vi "Autonomous Independent.vi"() -> ()   [LabVIEW 2012]
doc: "This VI is called when autonomous begins, and will automatically be terminated when autonomous ends. You can carry out timed or sensor driven robot movement independently without needing to return to the caller."
uses:
  <vilib>/Rock Robotics/WPI/RobotDrive/WPI_RobotDriveGetSetRefNum.vi
  Robot Global Data.vi
panel:
  out "Shooter Angle Good":bool
  out "Shooter Angle":T1(ring)
  out "Shooter Speed":T2(ring)
  out "Stop Drive":bool
  out "Shift Low":bool
  out "Feeder Happy":bool
  out "Auton Done":bool
  out "Shooter Happy":bool
  out "Shoot!":bool
  out "Delay Switch":u32
  out "Seccond Switch":u32
  out "First Switch":u32
  # "Be sure to right-click and choose Data Operations>>Make Current Value default if you want to save the array values with the VI"
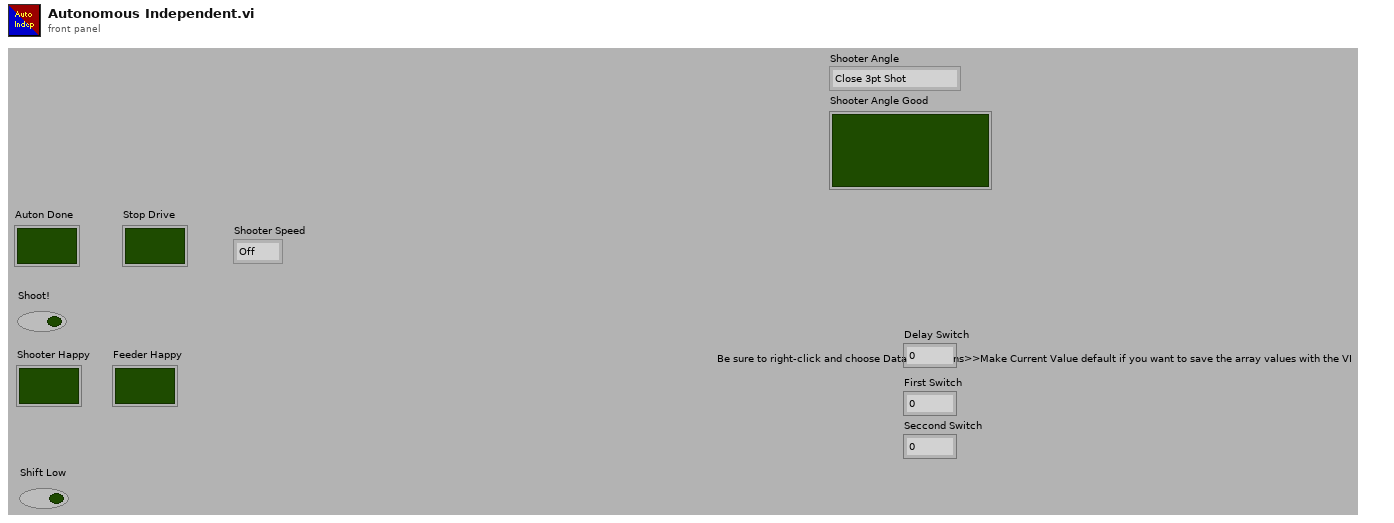
[diagram p1: front panel]
types:
  T1 = enum16{"Close 3pt Shot", "Far 3pt Shot", "Feeding"}
  T2 = enum16{"Off", "Close Pyramid 3pt", "Far Pyramid 3pt", "Feeder Shot", "UD Far 3pt Shot"}
  T3 = enum16{"Off", "Close Pyramid 3pt", "Far Pyramid 3pt", "Feeder Shot"}
  T4 = typedef "WPI_RobotDriveDevRef.ctl" = cluster{"DevStatus":errorcluster, "Motors[]":T5[], "Square Inputs":bool, "Max Output":dbl, "Isochronous":bool}
  T5 = typedef "WPI_MotorControlDeviceRef.ctl" = cluster{"DeviceStatus":errorcluster, "Type":enum16{"PWM", "CAN"}, "PWM":cluster{"Digital Module":T6, "PWM Channel":T7, "DeadBand":T8}, "CAN":cluster{"Device Number":u8, "Control Mode":T9, "Semaphore":T10, "Max Vout":dbl}, "Invert":bool, "TransformRef":T11, "InvTransformRef":T11}
  T6 = typedef "FPGA_TypedefDigitalModule.ctl" = enum16{"Digital Module 1", "Digital Module 2"}
  T7 = typedef "FPGA_DIOPWMChannel.ctl" = enum8{"PWM 1", "PWM 2", "PWM 3", "PWM 4", "PWM 5", "PWM 6", "PWM 7", "PWM 8", "PWM 9", "PWM 10", "Invalid"}
  T8 = typedef "WPI_PWMDeadband.ctl" = cluster{"Name":string, "maxPositivePwm":i32, "minPositivePwm":i32, "centerPwm":i32, "maxNegativePwm":i32, "minNegativePwm":i32, "angularRange":u16}
  T9 = typedef "WPI_CANJaguar_ControlMode.ctl" = enum8{"Percent VBus", "Current", "Speed", "Position", "Voltage"}
  T10 = typedef "Semaphore RefNum" = refnum<k1>
  T11 = typedef "WPI_PWMTransform_ConPane.ctl" = refnum<vi>
  T12 = typedef "WPI_GyroDevRef.ctl" = cluster{"DevStatus":errorcluster, "Analog Module":T13, "Analog Channel":T14, "Offset":dbl, "Gain (VoltsPerDegree/Second)":dbl}
  T13 = typedef "FPGA_TypedefAnalogModule.ctl" = enum16{"Analog Module 1", "Analog Module 2"}
  T14 = typedef "FPGA_AIChannel.ctl" = enum8{"AI 1", "AI 2", "AI 3", "AI 4", "AI 5", "AI 6", "AI 7", "AI 8", "Invalid"}
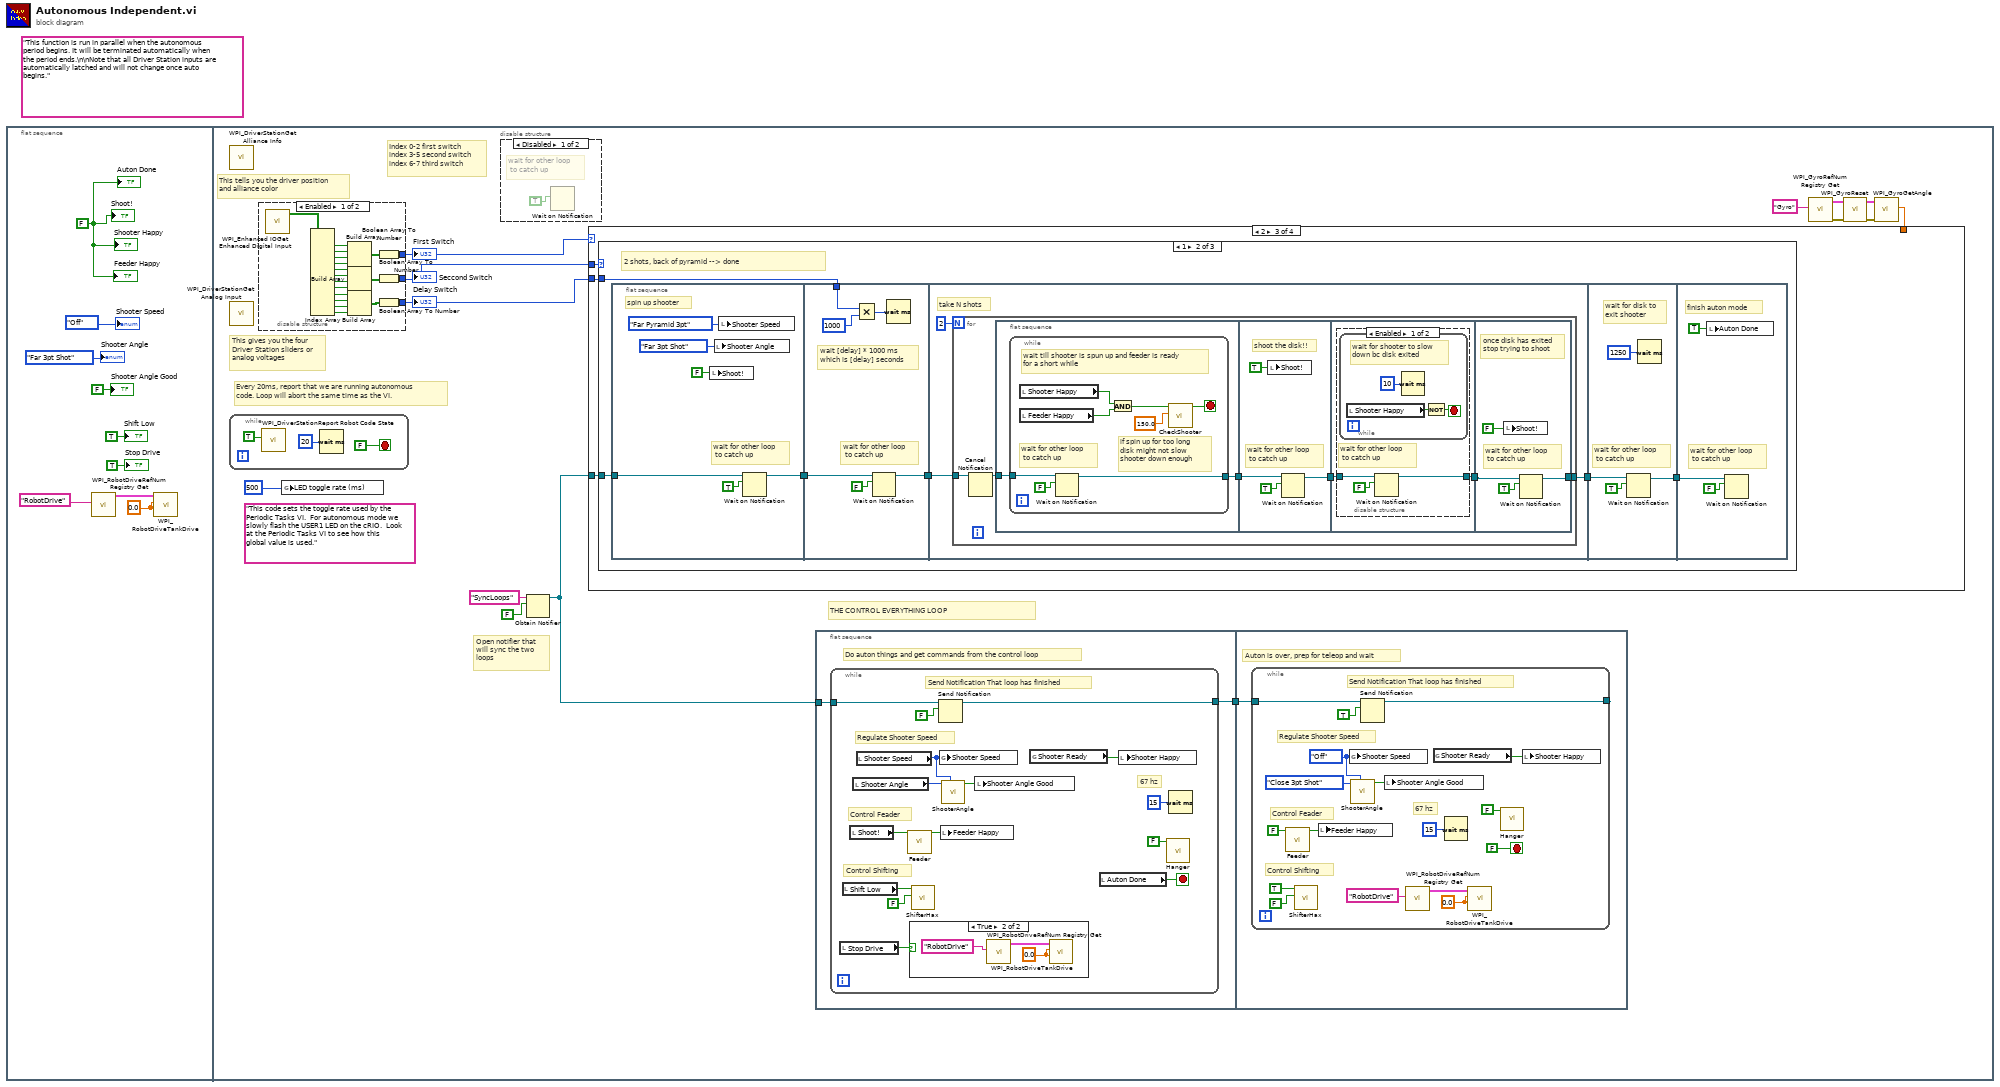
[diagram p0: block diagram]
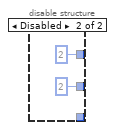
[diagram p2: hidden frame]
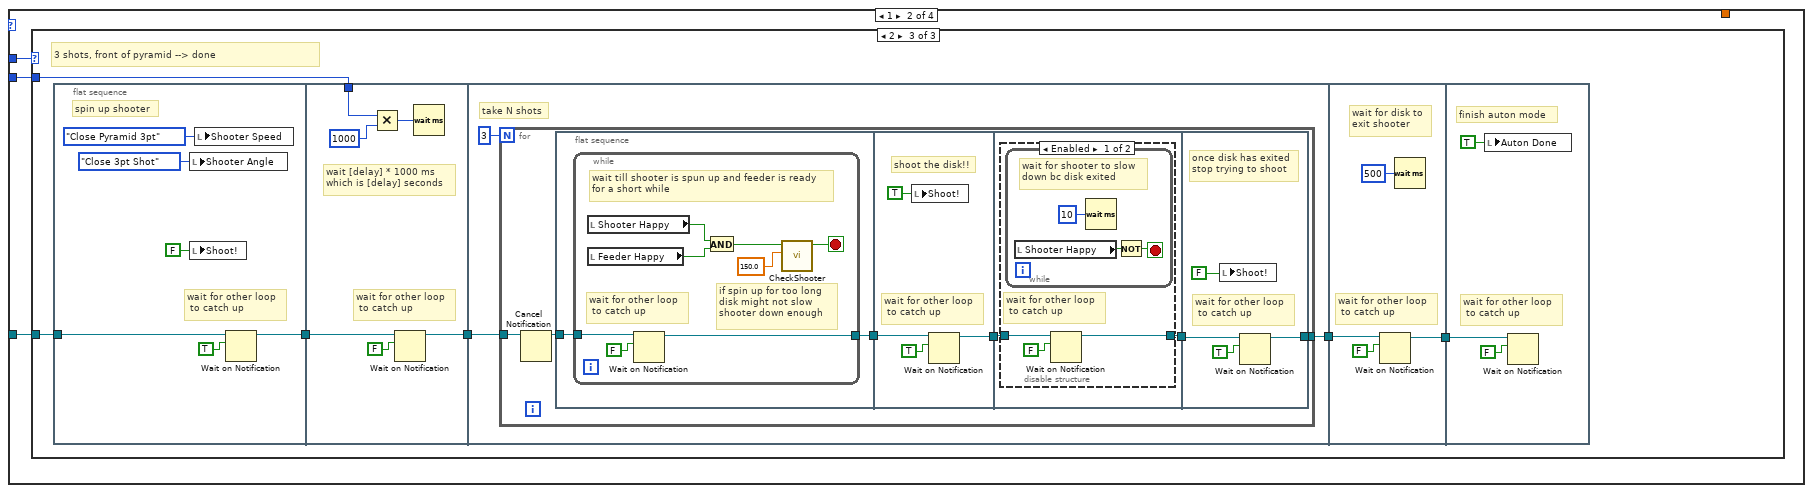
[diagram p6: hidden frame]
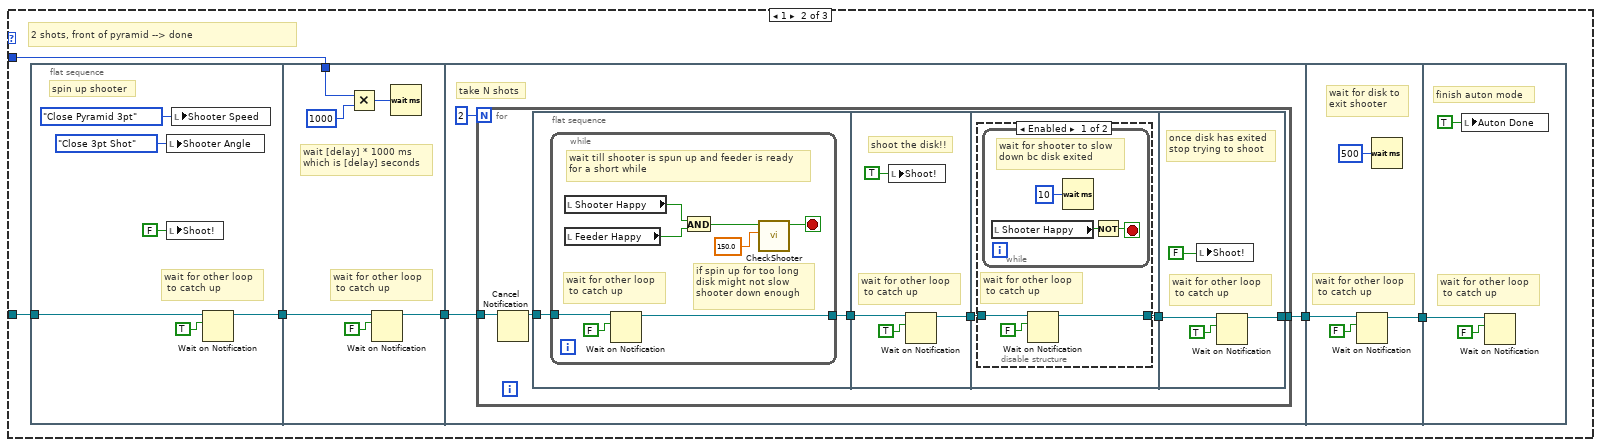
[diagram p8: hidden frame]
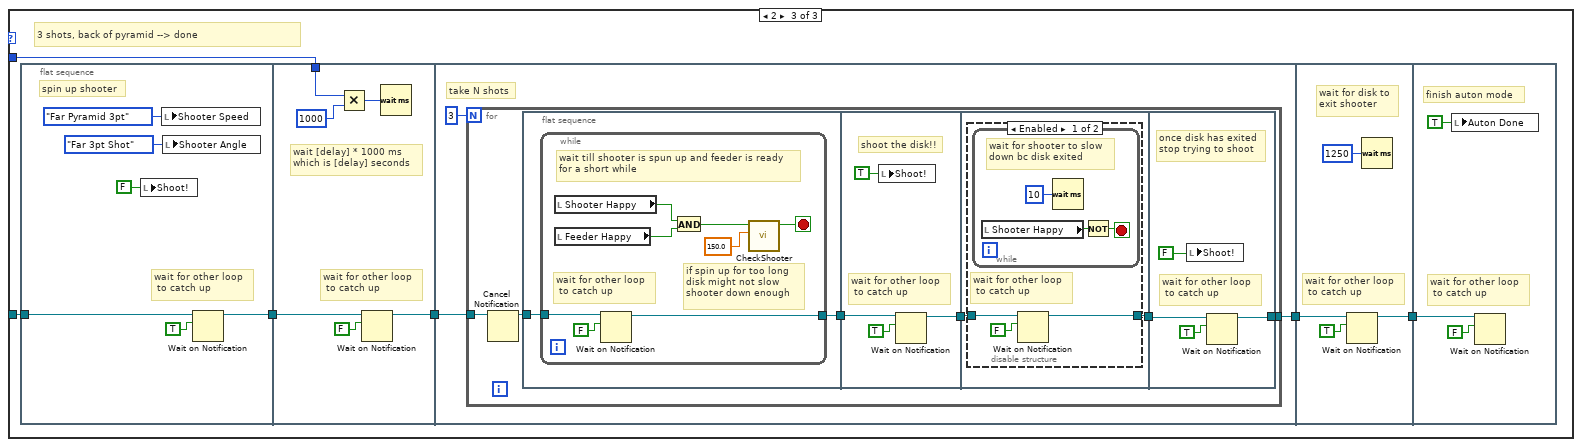
[diagram p13: hidden frame]
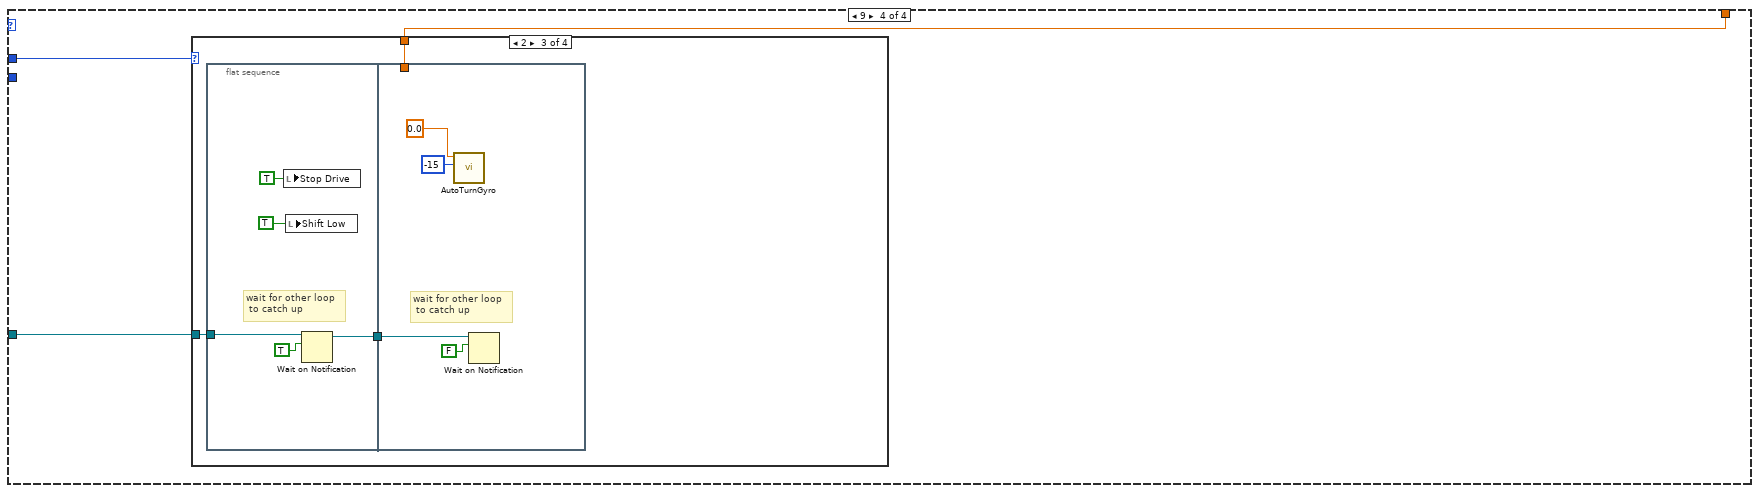
[diagram p15: hidden frame]
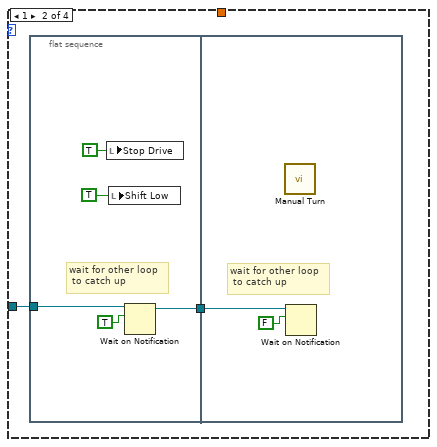
[diagram p17: hidden frame]
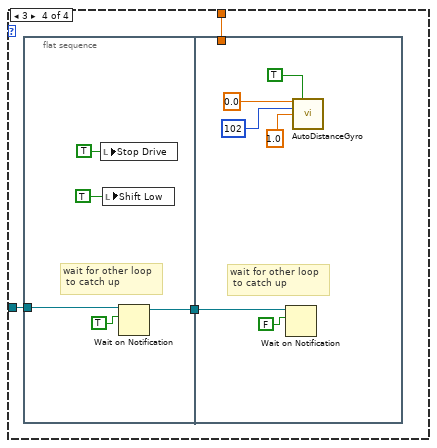
[diagram p18: hidden frame]
diagram:
  (unwired) "This function is run in parallel when the autonomous period begins. It will be terminated automatically when the period ends.\n\nNote that all Driver Station inputs are automatically latched and will not change once auto begins."
  n1 = flat-sequence {
    frame #0 {
      w5 = 0.0 ("Left axis value")
      w9 = FALSE
      n2 = call <vilib>:"WPI_RobotDriveRefNum Registry Get.vi"("refnum name"="RobotDrive") -> ("RobotDriveDevRef"=w6:T4)  [unwired: 1 in, 9 out]
      n3 = call <vilib>:"WPI_RobotDriveTankDrive.vi"("Right axis value"=w5, "Left axis value"=w5, "RobotDriveDevRef"=w6) -> ()  [unwired: 6 in, 3 out]
      "Feeder Happy" <- w9
      "Shift Low" <- TRUE ("Shift Low")
      "Stop Drive" <- TRUE ("Stop Drive")
      "Shoot!" <- w9
      "Shooter Happy" <- w9
      "Auton Done" <- w9
      "Shooter Speed" <- T3."Off" ("Shooter Speed")
      "Shooter Angle" <- T1."Far 3pt Shot" ("Target Shooter Angle")
      "Shooter Angle Good" <- FALSE ("Shooter Angle Good")
    }
    frame #1 {
      (unwired) "This code sets the toggle rate used by the Periodic Tasks VI.  For autonomous mode we slowly flash the USER1 LED on the cRIO.  Look at the Periodic Tasks VI to see how this global value is used."
      # "THE CONTROL EVERYTHING LOOP"
      # "Index 0-2 first switch\nindex 3-5 second switch\nindex 6-7 third switch"
      # "Open notifier that\nwill sync the two\nloops"
      # "Every 20ms, report that we are running autonomous\ncode. Loop will abort the same time as the VI."
      # "This tells you the driver position\nand alliance color"
      # "This gives you the four\nDriver Station sliders or\nanalog voltages"
      n4 = call <vilib>:"WPI_DriverStationGet Alliance Info.vi"() -> ()  [unwired: 12 out]
      n5 = call <vilib>:"WPI_DriverStationGet Analog Input.vi"() -> ()  [unwired: 12 out]
      n6 = while {
        stop <- FALSE stop-if-true
        n7 = call <vilib>:"WPI_DriverStationReport Robot Code State.vi"("Autonomous"=TRUE) -> ()  [unwired: 10 in, 1 out]
        n8 = Wait (ms)(milliseconds to wait=u32 20) -> ()  [unwired: 1 out]
      }
      n9 = disable-structure shown="Enabled" {
        disable-tunnel: [w26 u32 2 ("First Switch")] -> w18
        disable-tunnel: [w25 u32 2 ("Seccond Switch")] -> w17
        disable-tunnel: [w24 _] -> w15
        frame Enabled {
          n10 = call <vilib>:"WPI_Enhanced IOGet Enhanced Digital Input.vi"() -> ("Digital Input [1-16]"=w27:bool[])  [unwired: 10 in, 1 out]
          n11 = Index Array(array=w27) -> (element #1=w42:bool, element #2=w41:bool, element #3=w40:bool, element #4=w33:bool, element #5=w39:bool, element #6=w38:bool, element #7=w35:bool, element #8=w34:bool, element #9=w32:bool, element #10=w31:bool, element #11=w30:bool, element #12=w29:bool)  [unwired: 12 in]
          n12 = Build Array(w42, w41, w40, w33) -> (w36:bool[])
          n13 = Build Array(w39, w38, w35, w34) -> (w37:bool[])
          n14 = Build Array(w32, w31, w30, w29) -> (w28:bool[])
          n15 = Boolean Array To Number(Boolean array=w36) -> (number=w26:u32)
          n16 = Boolean Array To Number(Boolean array=w37) -> (number=w25:u32)
          n17 = Boolean Array To Number(Boolean array=w28) -> (number=w24:u32)
        }
        frame Disabled {
        }
      }
      "First Switch" <- w18
      "Seccond Switch" <- w17
      "Delay Switch" <- w15
      n18 = global write "Robot Global Data.vi" "LED toggle rate (ms)"(u32 500 ("LED ms toggle rate")) -> ()
      n19 = disable-structure shown="Disabled" {
        frame Disabled {
          # "wait for other loop\n to catch up"
          n20 = Wait on Notification(ignore previous (F)=TRUE) -> (notifier=w46:refnum<notifier>)  [unwired: 2 in, 4 out]
        }
        frame Enabled {
        }
      }
      n21 = Obtain Notifier(name (unnamed)="SyncLoops", notification data type=FALSE) -> (notifier out=w16:refnum<notifier>)  [unwired: 2 in, 2 out]
      n22 = flat-sequence {
        tunnel: w16 -> [w48]
        tunnel: [w47] -> w23
        tunnel: w23 -> [w67]
        frame #0 {
          # "Do auton things and get commands from the control loop"
          n23 = while {
            tunnel: w48 -> [w61]
            tunnel: [w59] -> w47
            stop <- w63 stop-if-true
            # "Regulate Shooter Speed"
            # "67 hz"
            # "Control Shifting"
            # "Control Feader"
            # "Send Notification That loop has finished"
            n24 = local read "Stop Drive"() -> (w57:bool)
            n25 = local read "Shift Low"() -> (w55:bool)
            n26 = local read "Shoot!"() -> (w53:bool)
            n27 = local read "Shooter Angle"() -> (w52:T1)
            n28 = local read "Shooter Speed"() -> (w51:T2)
            n29 = call "Feeder.vi"("SHOOT Button"=w53) -> ("Ready To Shoot?"=w60:bool)  [unwired: 10 in]
            n30 = case shown="True" w57 {
              frame False {
              }
              frame True {
                w66 = 0.0 ("Left axis value")
                n31 = call <vilib>:"WPI_RobotDriveRefNum Registry Get.vi"("refnum name"="RobotDrive") -> ("RobotDriveDevRef"=w65:T4)  [unwired: 1 in, 9 out]
                n32 = call <vilib>:"WPI_RobotDriveTankDrive.vi"("Right axis value"=w66, "Left axis value"=w66, "RobotDriveDevRef"=w65) -> ()  [unwired: 6 in, 3 out]
              }
            }
            n33 = call "ShifterHax.vi"("Automatic Shifting"=FALSE, "Manual Shift Low"=w55) -> ()  [unwired: 10 in]
            n34 = Send Notification(notification=FALSE, notifier=w61) -> (notifier out=w59:refnum<notifier>)  [unwired: 1 in, 1 out]
            n35 = global write "Robot Global Data.vi" "Shooter Speed"(w51) -> ()
            n36 = local write "Feeder Happy"(w60) -> ()
            n37 = call "ShooterAngle.vi"("Shooter Speed"=w51, "Target Shooter Angle"=w52) -> ("Shooter Angle Good"=w50:bool)  [unwired: 8 in, 1 out]
            n38 = local write "Shooter Angle Good"(w50) -> ()
            n39 = global read "Robot Global Data.vi" "Shooter Ready"() -> (w56:bool)
            n40 = local read "Auton Done"() -> (w63:bool)
            n41 = local write "Shooter Happy"(w56) -> ()
            n42 = call "Hanger.vi"("Hanger Up"=FALSE) -> ()  [unwired: 10 in, 1 out]
            n43 = Wait (ms)(milliseconds to wait=u32 15) -> ()  [unwired: 1 out]
          }
        }
        frame #1 {
          # "Auton is over, prep for teleop and wait"
          n44 = while {
            tunnel: w67 -> [w83]
            tunnel: [w81] -> _
            stop <- FALSE stop-if-true
            w77 = T2."Off" ("Shooter Speed")
            w75 = 0.0 ("Left axis value")
            # "Regulate Shooter Speed"
            # "67 hz"
            # "Control Shifting"
            # "Control Feader"
            # "Send Notification That loop has finished"
            n45 = call "Feeder.vi"("SHOOT Button"=FALSE) -> ("Ready To Shoot?"=w82:bool)  [unwired: 10 in]
            n46 = call "ShifterHax.vi"("Automatic Shifting"=FALSE, "Manual Shift Low"=TRUE) -> ()  [unwired: 10 in]
            n47 = local write "Feeder Happy"(w82) -> ()
            n48 = global write "Robot Global Data.vi" "Shooter Speed"(w77) -> ()
            n49 = call "ShooterAngle.vi"("Shooter Speed"=w77, "Target Shooter Angle"=T1."Close 3pt Shot") -> ("Shooter Angle Good"=w76:bool)  [unwired: 8 in, 1 out]
            n50 = Send Notification(notification=TRUE, notifier=w83) -> (notifier out=w81:refnum<notifier>)  [unwired: 1 in, 1 out]
            n51 = local write "Shooter Angle Good"(w76) -> ()
            n52 = call <vilib>:"WPI_RobotDriveRefNum Registry Get.vi"("refnum name"="RobotDrive") -> ("RobotDriveDevRef"=w74:T4)  [unwired: 1 in, 9 out]
            n53 = global read "Robot Global Data.vi" "Shooter Ready"() -> (w79:bool)
            n54 = Wait (ms)(milliseconds to wait=u32 15) -> ()  [unwired: 1 out]
            n55 = call <vilib>:"WPI_RobotDriveTankDrive.vi"("Right axis value"=w75, "Left axis value"=w75, "RobotDriveDevRef"=w74) -> ()  [unwired: 6 in, 3 out]
            n56 = call "Hanger.vi"("Hanger Up"=FALSE) -> ()  [unwired: 10 in, 1 out]
            n57 = local write "Shooter Happy"(w79) -> ()
          }
        }
      }
      n58 = call <vilib>:"WPI_GyroRefNum Registry Get.vi"("refnum name"="Gyro") -> ("error out"=w14:errorcluster, "GyroDevRef"=w13:T12)  [unwired: 9 in]
      n59 = call <vilib>:"WPI_GyroReset.vi"("error in (no error)"=w14, "GyroDevRef"=w13) -> ("error out"=w12:errorcluster, "GyroDevRef"=w11:T12)  [unwired: 8 in]
      n60 = call <vilib>:"WPI_GyroGetAngle.vi"("error in (no error)"=w12, "GyroDevRef"=w11) -> ("Angle"=w10:dbl)  [unwired: 6 in, 3 out]
      n61 = case shown="2" w18 {
        tunnel: w17 -> [_ w87 w210 w333]
        tunnel: w16 -> [_ w86 w209 w332]
        tunnel: w15 -> [_ w85 w208 _]
        tunnel: w10 -> [_ _ _ w331]
        frame 0, Default {
          # "do nothing"
        }
        frame 1 {
          n62 = case shown="2" w87 {
            tunnel: w86 -> [_ w90 w150]
            tunnel: w85 -> [_ w93 w153]
            frame 0, Default {
              # "do nothing"
            }
            frame 1 {
              # "2 shots, front of pyramid --> done"
              n63 = flat-sequence {
                tunnel: [w98] -> w92
                tunnel: w90 -> [w97]
                tunnel: w93 -> [w103]
                tunnel: w92 -> [w101]
                tunnel: [w100] -> w91
                tunnel: w91 -> [w107]
                tunnel: [w106] -> w89
                tunnel: w89 -> [w142]
                tunnel: [w141] -> w88
                tunnel: w88 -> [w145]
                frame #0 {
                  # "wait for other loop\n to catch up"
                  # "spin up shooter"
                  n64 = local write "Shooter Angle"(T1."Close 3pt Shot" ("Shooter Angle")) -> ()
                  n65 = local write "Shoot!"(FALSE ("Shoot!")) -> ()
                  n66 = local write "Shooter Speed"(T3."Close Pyramid 3pt" ("Shooter Speed")) -> ()
                  n67 = Wait on Notification(notifier=w97, ignore previous (F)=TRUE) -> (notifier out=w98:refnum<notifier>)  [unwired: 2 in, 3 out]
                }
                frame #1 {
                  # "wait for other loop\n to catch up"
                  # "wait [delay] * 1000 ms\nwhich is [delay] seconds"
                  n68 = Multiply(x=w103, y=1000) -> (x*y=w105:u32)
                  n69 = Wait on Notification(notifier=w101, ignore previous (F)=FALSE) -> (notifier out=w100:refnum<notifier>)  [unwired: 2 in, 3 out]
                  n70 = Wait (ms)(milliseconds to wait=w105) -> ()  [unwired: 1 out]
                }
                frame #2 {
                  # "take N shots"
                  n71 = for {
                    N: 2 -> [_]
                    tunnel: w107 -> [w113]
                    tunnel: [w111] -> w106
                    n72 = Cancel Notification(0:w113) -> (8:w114:refnum<notifier>)  [unwired: 1 in, 2 out]
                    n73 = flat-sequence {
                      tunnel: w114 -> [w116]
                      tunnel: [w115] -> w112
                      tunnel: w112 -> [w126]
                      tunnel: [w125] -> w110
                      tunnel: w110 -> [w129]
                      tunnel: [w130] -> w109
                      tunnel: [w139] -> w111
                      tunnel: w109 -> [w138]
                      frame #0 {
                        n74 = while {
                          tunnel: w116 -> [w118]
                          tunnel: [w117] -> w115
                          stop <- w120 stop-if-true
                          # "if spin up for too long\ndisk might not slow\nshooter down enough"
                          # "wait for other loop\n to catch up"
                          # "wait till shooter is spun up and feeder is ready\nfor a short while"
                          n75 = local read "Shooter Happy"() -> (w123:bool)
                          n76 = local read "Feeder Happy"() -> (w122:bool)
                          n77 = Wait on Notification(notifier=w118, ignore previous (F)=FALSE) -> (notifier out=w117:refnum<notifier>)  [unwired: 2 in, 3 out]
                          n78 = And(x=w123, y=w122) -> (x .and. y?=w121:bool)
                          n79 = call "CheckShooter.vi"("Time for happy (ms)"=150.0, "Shooter Good?"=w121) -> ("Good to shoot"=w120:bool)  [unwired: 9 in]
                        }
                      }
                      frame #1 {
                        # "wait for other loop\n to catch up"
                        # "shoot the disk!!"
                        n80 = local write "Shoot!"(TRUE ("Shoot!")) -> ()
                        n81 = Wait on Notification(notifier=w126, ignore previous (F)=TRUE) -> (notifier out=w125:refnum<notifier>)  [unwired: 2 in, 3 out]
                      }
                      frame #2 {
                        n82 = disable-structure shown="Enabled" {
                          disable-tunnel: [w132 _] -> w130
                          disable-tunnel: w129 -> [w131 _]
                          frame Enabled {
                            # "wait for other loop\n to catch up"
                            n83 = while {
                              stop <- w136 stop-if-true
                              # "wait for shooter to slow\ndown bc disk exited"
                              n84 = local read "Shooter Happy"() -> (w135:bool)
                              n85 = Wait (ms)(milliseconds to wait=u32 10) -> ()  [unwired: 1 out]
                              n86 = Not(x=w135) -> (.not. x?=w136:bool)
                            }
                            n87 = Wait on Notification(notifier=w131, ignore previous (F)=FALSE) -> (notifier out=w132:refnum<notifier>)  [unwired: 2 in, 3 out]
                          }
                          frame Disabled {
                          }
                        }
                      }
                      frame #3 {
                        # "once disk has exited\nstop trying to shoot"
                        # "wait for other loop\n to catch up"
                        n88 = local write "Shoot!"(FALSE) -> ()
                        n89 = Wait on Notification(notifier=w138, ignore previous (F)=TRUE) -> (notifier out=w139:refnum<notifier>)  [unwired: 2 in, 3 out]
                      }
                    }
                  }
                }
                frame #3 {
                  # "wait for other loop\n to catch up"
                  # "wait for disk to\nexit shooter"
                  n90 = Wait on Notification(notifier=w142, ignore previous (F)=FALSE) -> (notifier out=w141:refnum<notifier>)  [unwired: 2 in, 3 out]
                  n91 = Wait (ms)(milliseconds to wait=u32 500) -> ()  [unwired: 1 out]
                }
                frame #4 {
                  # "wait for other loop\n to catch up"
                  # "finish auton mode"
                  n92 = local write "Auton Done"(TRUE ("Auton Done")) -> ()
                  n93 = Wait on Notification(notifier=w145, ignore previous (F)=FALSE) -> ()  [unwired: 2 in, 4 out]
                }
              }
            }
            frame 2 {
              # "3 shots, front of pyramid --> done"
              n94 = flat-sequence {
                tunnel: [w158] -> w152
                tunnel: w150 -> [w157]
                tunnel: w153 -> [w163]
                tunnel: w152 -> [w161]
                tunnel: [w160] -> w151
                tunnel: w151 -> [w167]
                tunnel: [w166] -> w149
                tunnel: w149 -> [w202]
                tunnel: [w201] -> w148
                tunnel: w148 -> [w205]
                frame #0 {
                  # "wait for other loop\n to catch up"
                  # "spin up shooter"
                  n95 = local write "Shooter Angle"(T1."Close 3pt Shot" ("Shooter Angle")) -> ()
                  n96 = local write "Shoot!"(FALSE ("Shoot!")) -> ()
                  n97 = local write "Shooter Speed"(T3."Close Pyramid 3pt" ("Shooter Speed")) -> ()
                  n98 = Wait on Notification(notifier=w157, ignore previous (F)=TRUE) -> (notifier out=w158:refnum<notifier>)  [unwired: 2 in, 3 out]
                }
                frame #1 {
                  # "wait for other loop\n to catch up"
                  # "wait [delay] * 1000 ms\nwhich is [delay] seconds"
                  n99 = Multiply(x=w163, y=1000) -> (x*y=w165:u32)
                  n100 = Wait on Notification(notifier=w161, ignore previous (F)=FALSE) -> (notifier out=w160:refnum<notifier>)  [unwired: 2 in, 3 out]
                  n101 = Wait (ms)(milliseconds to wait=w165) -> ()  [unwired: 1 out]
                }
                frame #2 {
                  # "take N shots"
                  n102 = for {
                    N: 3 -> [_]
                    tunnel: w167 -> [w173]
                    tunnel: [w171] -> w166
                    n103 = Cancel Notification(0:w173) -> (8:w174:refnum<notifier>)  [unwired: 1 in, 2 out]
                    n104 = flat-sequence {
                      tunnel: w174 -> [w176]
                      tunnel: [w175] -> w172
                      tunnel: w172 -> [w186]
                      tunnel: [w185] -> w170
                      tunnel: w170 -> [w189]
                      tunnel: [w190] -> w169
                      tunnel: [w199] -> w171
                      tunnel: w169 -> [w198]
                      frame #0 {
                        n105 = while {
                          tunnel: w176 -> [w178]
                          tunnel: [w177] -> w175
                          stop <- w180 stop-if-true
                          # "if spin up for too long\ndisk might not slow\nshooter down enough"
                          # "wait for other loop\n to catch up"
                          # "wait till shooter is spun up and feeder is ready\nfor a short while"
                          n106 = local read "Shooter Happy"() -> (w183:bool)
                          n107 = local read "Feeder Happy"() -> (w182:bool)
                          n108 = Wait on Notification(notifier=w178, ignore previous (F)=FALSE) -> (notifier out=w177:refnum<notifier>)  [unwired: 2 in, 3 out]
                          n109 = And(x=w183, y=w182) -> (x .and. y?=w181:bool)
                          n110 = call "CheckShooter.vi"("Time for happy (ms)"=150.0, "Shooter Good?"=w181) -> ("Good to shoot"=w180:bool)  [unwired: 9 in]
                        }
                      }
                      frame #1 {
                        # "wait for other loop\n to catch up"
                        # "shoot the disk!!"
                        n111 = local write "Shoot!"(TRUE ("Shoot!")) -> ()
                        n112 = Wait on Notification(notifier=w186, ignore previous (F)=TRUE) -> (notifier out=w185:refnum<notifier>)  [unwired: 2 in, 3 out]
                      }
                      frame #2 {
                        n113 = disable-structure shown="Enabled" {
                          disable-tunnel: [w192 _] -> w190
                          disable-tunnel: w189 -> [w191 _]
                          frame Enabled {
                            # "wait for other loop\n to catch up"
                            n114 = while {
                              stop <- w196 stop-if-true
                              # "wait for shooter to slow\ndown bc disk exited"
                              n115 = local read "Shooter Happy"() -> (w195:bool)
                              n116 = Wait (ms)(milliseconds to wait=u32 10) -> ()  [unwired: 1 out]
                              n117 = Not(x=w195) -> (.not. x?=w196:bool)
                            }
                            n118 = Wait on Notification(notifier=w191, ignore previous (F)=FALSE) -> (notifier out=w192:refnum<notifier>)  [unwired: 2 in, 3 out]
                          }
                          frame Disabled {
                          }
                        }
                      }
                      frame #3 {
                        # "once disk has exited\nstop trying to shoot"
                        # "wait for other loop\n to catch up"
                        n119 = local write "Shoot!"(FALSE) -> ()
                        n120 = Wait on Notification(notifier=w198, ignore previous (F)=TRUE) -> (notifier out=w199:refnum<notifier>)  [unwired: 2 in, 3 out]
                      }
                    }
                  }
                }
                frame #3 {
                  # "wait for other loop\n to catch up"
                  # "wait for disk to\nexit shooter"
                  n121 = Wait on Notification(notifier=w202, ignore previous (F)=FALSE) -> (notifier out=w201:refnum<notifier>)  [unwired: 2 in, 3 out]
                  n122 = Wait (ms)(milliseconds to wait=u32 500) -> ()  [unwired: 1 out]
                }
                frame #4 {
                  # "wait for other loop\n to catch up"
                  # "finish auton mode"
                  n123 = local write "Auton Done"(TRUE ("Auton Done")) -> ()
                  n124 = Wait on Notification(notifier=w205, ignore previous (F)=FALSE) -> ()  [unwired: 2 in, 4 out]
                }
              }
            }
          }
        }
        frame 2 {
          n125 = case shown="1" w210 {
            tunnel: w209 -> [_ w213 w273]
            tunnel: w208 -> [_ w216 w276]
            frame 0, Default {
              # "do nothing"
            }
            frame 1 {
              # "2 shots, back of pyramid --> done"
              n126 = flat-sequence {
                tunnel: [w221] -> w215
                tunnel: w213 -> [w220]
                tunnel: w216 -> [w226]
                tunnel: w215 -> [w224]
                tunnel: [w223] -> w214
                tunnel: w214 -> [w230]
                tunnel: [w229] -> w212
                tunnel: w212 -> [w265]
                tunnel: [w264] -> w211
                tunnel: w211 -> [w268]
                frame #0 {
                  # "wait for other loop\n to catch up"
                  # "spin up shooter"
                  n127 = local write "Shoot!"(FALSE ("Shoot!")) -> ()
                  n128 = local write "Shooter Angle"(T1."Far 3pt Shot" ("Shooter Angle")) -> ()
                  n129 = local write "Shooter Speed"(T2."Far Pyramid 3pt" ("Shooter Speed")) -> ()
                  n130 = Wait on Notification(notifier=w220, ignore previous (F)=TRUE) -> (notifier out=w221:refnum<notifier>)  [unwired: 2 in, 3 out]
                }
                frame #1 {
                  # "wait for other loop\n to catch up"
                  # "wait [delay] * 1000 ms\nwhich is [delay] seconds"
                  n131 = Multiply(x=w226, y=1000) -> (x*y=w228:u32)
                  n132 = Wait on Notification(notifier=w224, ignore previous (F)=FALSE) -> (notifier out=w223:refnum<notifier>)  [unwired: 2 in, 3 out]
                  n133 = Wait (ms)(milliseconds to wait=w228) -> ()  [unwired: 1 out]
                }
                frame #2 {
                  # "take N shots"
                  n134 = for {
                    N: 2 -> [_]
                    tunnel: w230 -> [w236]
                    tunnel: [w234] -> w229
                    n135 = Cancel Notification(0:w236) -> (8:w237:refnum<notifier>)  [unwired: 1 in, 2 out]
                    n136 = flat-sequence {
                      tunnel: w237 -> [w239]
                      tunnel: [w238] -> w235
                      tunnel: w235 -> [w249]
                      tunnel: [w248] -> w233
                      tunnel: w233 -> [w252]
                      tunnel: [w253] -> w232
                      tunnel: [w262] -> w234
                      tunnel: w232 -> [w261]
                      frame #0 {
                        n137 = while {
                          tunnel: w239 -> [w241]
                          tunnel: [w240] -> w238
                          stop <- w243 stop-if-true
                          # "if spin up for too long\ndisk might not slow\nshooter down enough"
                          # "wait for other loop\n to catch up"
                          # "wait till shooter is spun up and feeder is ready\nfor a short while"
                          n138 = local read "Shooter Happy"() -> (w246:bool)
                          n139 = local read "Feeder Happy"() -> (w245:bool)
                          n140 = Wait on Notification(notifier=w241, ignore previous (F)=FALSE) -> (notifier out=w240:refnum<notifier>)  [unwired: 2 in, 3 out]
                          n141 = And(x=w246, y=w245) -> (x .and. y?=w244:bool)
                          n142 = call "CheckShooter.vi"("Time for happy (ms)"=150.0, "Shooter Good?"=w244) -> ("Good to shoot"=w243:bool)  [unwired: 9 in]
                        }
                      }
                      frame #1 {
                        # "wait for other loop\n to catch up"
                        # "shoot the disk!!"
                        n143 = local write "Shoot!"(TRUE ("Shoot!")) -> ()
                        n144 = Wait on Notification(notifier=w249, ignore previous (F)=TRUE) -> (notifier out=w248:refnum<notifier>)  [unwired: 2 in, 3 out]
                      }
                      frame #2 {
                        n145 = disable-structure shown="Enabled" {
                          disable-tunnel: [w255 _] -> w253
                          disable-tunnel: w252 -> [w254 _]
                          frame Enabled {
                            # "wait for other loop\n to catch up"
                            n146 = while {
                              stop <- w259 stop-if-true
                              # "wait for shooter to slow\ndown bc disk exited"
                              n147 = local read "Shooter Happy"() -> (w258:bool)
                              n148 = Wait (ms)(milliseconds to wait=u32 10) -> ()  [unwired: 1 out]
                              n149 = Not(x=w258) -> (.not. x?=w259:bool)
                            }
                            n150 = Wait on Notification(notifier=w254, ignore previous (F)=FALSE) -> (notifier out=w255:refnum<notifier>)  [unwired: 2 in, 3 out]
                          }
                          frame Disabled {
                          }
                        }
                      }
                      frame #3 {
                        # "once disk has exited\nstop trying to shoot"
                        # "wait for other loop\n to catch up"
                        n151 = local write "Shoot!"(FALSE) -> ()
                        n152 = Wait on Notification(notifier=w261, ignore previous (F)=TRUE) -> (notifier out=w262:refnum<notifier>)  [unwired: 2 in, 3 out]
                      }
                    }
                  }
                }
                frame #3 {
                  # "wait for other loop\n to catch up"
                  # "wait for disk to\nexit shooter"
                  n153 = Wait on Notification(notifier=w265, ignore previous (F)=TRUE) -> (notifier out=w264:refnum<notifier>)  [unwired: 2 in, 3 out]
                  n154 = Wait (ms)(milliseconds to wait=u32 1250) -> ()  [unwired: 1 out]
                }
                frame #4 {
                  # "wait for other loop\n to catch up"
                  # "finish auton mode"
                  n155 = local write "Auton Done"(TRUE ("Auton Done")) -> ()
                  n156 = Wait on Notification(notifier=w268, ignore previous (F)=FALSE) -> ()  [unwired: 2 in, 4 out]
                }
              }
            }
            frame 2 {
              # "3 shots, back of pyramid --> done"
              n157 = flat-sequence {
                tunnel: [w281] -> w275
                tunnel: w273 -> [w280]
                tunnel: w276 -> [w286]
                tunnel: w275 -> [w284]
                tunnel: [w283] -> w274
                tunnel: w274 -> [w290]
                tunnel: [w289] -> w272
                tunnel: w272 -> [w325]
                tunnel: [w324] -> w271
                tunnel: w271 -> [w328]
                frame #0 {
                  # "wait for other loop\n to catch up"
                  # "spin up shooter"
                  n158 = local write "Shoot!"(FALSE ("Shoot!")) -> ()
                  n159 = local write "Shooter Speed"(T2."Far Pyramid 3pt" ("Shooter Speed")) -> ()
                  n160 = local write "Shooter Angle"(T1."Far 3pt Shot" ("Shooter Angle")) -> ()
                  n161 = Wait on Notification(notifier=w280, ignore previous (F)=TRUE) -> (notifier out=w281:refnum<notifier>)  [unwired: 2 in, 3 out]
                }
                frame #1 {
                  # "wait for other loop\n to catch up"
                  # "wait [delay] * 1000 ms\nwhich is [delay] seconds"
                  n162 = Multiply(x=w286, y=1000) -> (x*y=w288:u32)
                  n163 = Wait on Notification(notifier=w284, ignore previous (F)=FALSE) -> (notifier out=w283:refnum<notifier>)  [unwired: 2 in, 3 out]
                  n164 = Wait (ms)(milliseconds to wait=w288) -> ()  [unwired: 1 out]
                }
                frame #2 {
                  # "take N shots"
                  n165 = for {
                    N: 3 -> [_]
                    tunnel: w290 -> [w296]
                    tunnel: [w294] -> w289
                    n166 = Cancel Notification(0:w296) -> (8:w297:refnum<notifier>)  [unwired: 1 in, 2 out]
                    n167 = flat-sequence {
                      tunnel: w297 -> [w299]
                      tunnel: [w298] -> w295
                      tunnel: w295 -> [w309]
                      tunnel: [w308] -> w293
                      tunnel: w293 -> [w312]
                      tunnel: [w313] -> w292
                      tunnel: [w322] -> w294
                      tunnel: w292 -> [w321]
                      frame #0 {
                        n168 = while {
                          tunnel: w299 -> [w301]
                          tunnel: [w300] -> w298
                          stop <- w303 stop-if-true
                          # "if spin up for too long\ndisk might not slow\nshooter down enough"
                          # "wait for other loop\n to catch up"
                          # "wait till shooter is spun up and feeder is ready\nfor a short while"
                          n169 = local read "Shooter Happy"() -> (w306:bool)
                          n170 = local read "Feeder Happy"() -> (w305:bool)
                          n171 = Wait on Notification(notifier=w301, ignore previous (F)=FALSE) -> (notifier out=w300:refnum<notifier>)  [unwired: 2 in, 3 out]
                          n172 = And(x=w306, y=w305) -> (x .and. y?=w304:bool)
                          n173 = call "CheckShooter.vi"("Time for happy (ms)"=150.0, "Shooter Good?"=w304) -> ("Good to shoot"=w303:bool)  [unwired: 9 in]
                        }
                      }
                      frame #1 {
                        # "wait for other loop\n to catch up"
                        # "shoot the disk!!"
                        n174 = local write "Shoot!"(TRUE ("Shoot!")) -> ()
                        n175 = Wait on Notification(notifier=w309, ignore previous (F)=TRUE) -> (notifier out=w308:refnum<notifier>)  [unwired: 2 in, 3 out]
                      }
                      frame #2 {
                        n176 = disable-structure shown="Enabled" {
                          disable-tunnel: [w315 _] -> w313
                          disable-tunnel: w312 -> [w314 _]
                          frame Enabled {
                            # "wait for other loop\n to catch up"
                            n177 = while {
                              stop <- w319 stop-if-true
                              # "wait for shooter to slow\ndown bc disk exited"
                              n178 = local read "Shooter Happy"() -> (w318:bool)
                              n179 = Wait (ms)(milliseconds to wait=u32 10) -> ()  [unwired: 1 out]
                              n180 = Not(x=w318) -> (.not. x?=w319:bool)
                            }
                            n181 = Wait on Notification(notifier=w314, ignore previous (F)=FALSE) -> (notifier out=w315:refnum<notifier>)  [unwired: 2 in, 3 out]
                          }
                          frame Disabled {
                          }
                        }
                      }
                      frame #3 {
                        # "once disk has exited\nstop trying to shoot"
                        # "wait for other loop\n to catch up"
                        n182 = local write "Shoot!"(FALSE) -> ()
                        n183 = Wait on Notification(notifier=w321, ignore previous (F)=TRUE) -> (notifier out=w322:refnum<notifier>)  [unwired: 2 in, 3 out]
                      }
                    }
                  }
                }
                frame #3 {
                  # "wait for other loop\n to catch up"
                  # "wait for disk to\nexit shooter"
                  n184 = Wait on Notification(notifier=w325, ignore previous (F)=TRUE) -> (notifier out=w324:refnum<notifier>)  [unwired: 2 in, 3 out]
                  n185 = Wait (ms)(milliseconds to wait=u32 1250) -> ()  [unwired: 1 out]
                }
                frame #4 {
                  # "wait for other loop\n to catch up"
                  # "finish auton mode"
                  n186 = local write "Auton Done"(TRUE ("Auton Done")) -> ()
                  n187 = Wait on Notification(notifier=w328, ignore previous (F)=FALSE) -> ()  [unwired: 2 in, 4 out]
                }
              }
            }
          }
        }
        frame 9 {
          n188 = case shown="2" w333 {
            tunnel: w332 -> [_ w335 w345 w357]
            tunnel: w331 -> [_ _ w343 w355]
            frame 0, Default {
            }
            frame 1 {
              n189 = flat-sequence {
                tunnel: w335 -> [w339]
                tunnel: [w338] -> w334
                tunnel: w334 -> [w341]
                frame #0 {
                  # "wait for other loop\n to catch up"
                  n190 = local write "Stop Drive"(TRUE ("Stop Drive")) -> ()
                  n191 = local write "Shift Low"(TRUE ("Stop Drive")) -> ()
                  n192 = Wait on Notification(notifier=w339, ignore previous (F)=TRUE) -> (notifier out=w338:refnum<notifier>)  [unwired: 2 in, 3 out]
                }
                frame #1 {
                  # "wait for other loop\n to catch up"
                  n193 = call "Manual Turn.vi"() -> ()  [unwired: 12 in]
                  n194 = Wait on Notification(notifier=w341, ignore previous (F)=FALSE) -> ()  [unwired: 2 in, 4 out]
                }
              }
            }
            frame 2 {
              n195 = flat-sequence {
                tunnel: w345 -> [w349]
                tunnel: [w348] -> w344
                tunnel: w344 -> [w353]
                tunnel: w343 -> [_]
                frame #0 {
                  # "wait for other loop\n to catch up"
                  n196 = local write "Stop Drive"(TRUE ("Stop Drive")) -> ()
                  n197 = local write "Shift Low"(TRUE ("Stop Drive")) -> ()
                  n198 = Wait on Notification(notifier=w349, ignore previous (F)=TRUE) -> (notifier out=w348:refnum<notifier>)  [unwired: 2 in, 3 out]
                }
                frame #1 {
                  # "wait for other loop\n to catch up"
                  n199 = call "AutoTurnGyro.vi"("Turn Amount"=-15, "Initial Angle"=0.0) -> ()  [unwired: 8 in, 2 out]
                  n200 = Wait on Notification(notifier=w353, ignore previous (F)=FALSE) -> ()  [unwired: 2 in, 4 out]
                }
              }
            }
            frame 3 {
              n201 = flat-sequence {
                tunnel: w357 -> [w361]
                tunnel: [w360] -> w356
                tunnel: w356 -> [w367]
                tunnel: w355 -> [_]
                frame #0 {
                  # "wait for other loop\n to catch up"
                  n202 = local write "Stop Drive"(TRUE ("Stop Drive")) -> ()
                  n203 = local write "Shift Low"(TRUE ("Stop Drive")) -> ()
                  n204 = Wait on Notification(notifier=w361, ignore previous (F)=TRUE) -> (notifier out=w360:refnum<notifier>)  [unwired: 2 in, 3 out]
                }
                frame #1 {
                  # "wait for other loop\n to catch up"
                  n205 = Wait on Notification(notifier=w367, ignore previous (F)=FALSE) -> ()  [unwired: 2 in, 4 out]
                  n206 = call "AutoDistanceGyro.vi"("InitialAngle"=0.0 ("Initial Angle"), "Reset Encoders"=TRUE, "TargetDistance"=102 ("Turn Amount"), "Motor Speed"=1.0) -> ()  [unwired: 10 in, 2 out]
                }
              }
            }
          }
        }
      }
    }
  }
